vi "EMV Cold Water Check.vi"(4 "T7_DELTA_INDICATING_FLOW":dbl, 6 "Cold Water Supply Temperature":dbl, 7 "T7 Detect?":bool, 8 "error in (no error)":errorcluster, 9 "T7_DELTA_FLOW_THRESHOLD":dbl, 11 "Current T7 Temperatures":dbl[](array[numeric])) -> (0 "error out":errorcluster, 3 "T7 Detect?":bool)   [LabVIEW 2020]
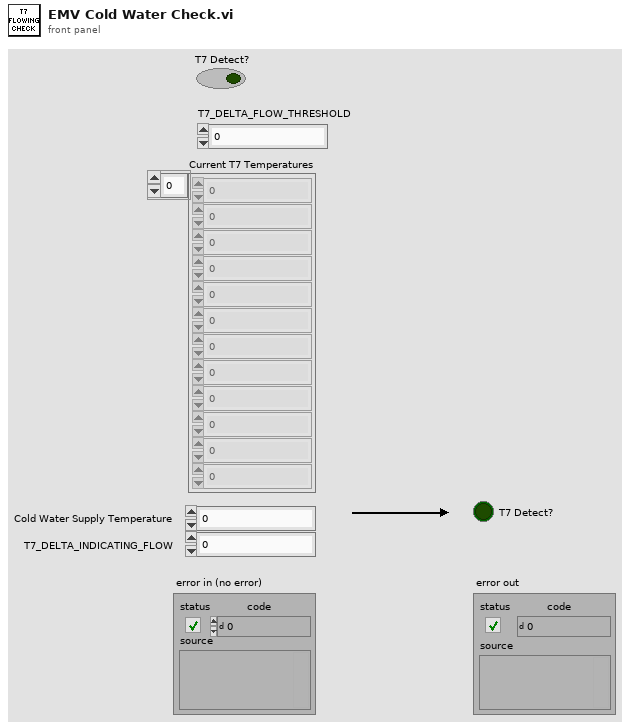
[diagram p1: front panel]
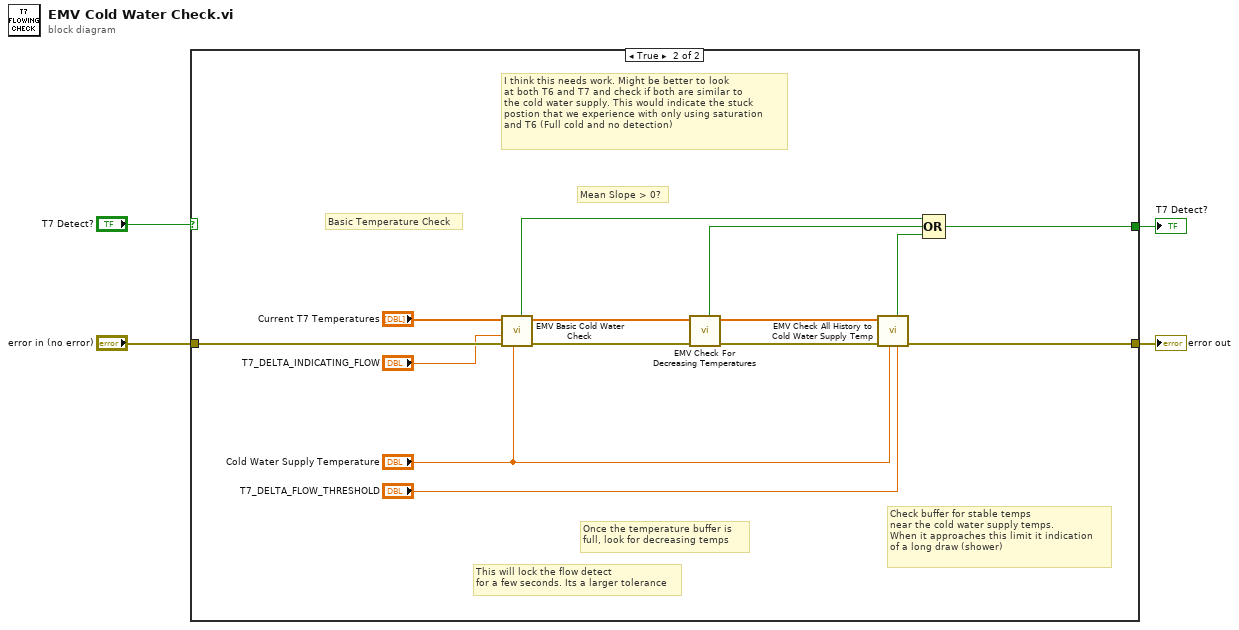
[diagram p0: block diagram]
diagram:
  n1 = case shown="True" "T7 Detect?" {
    selector: "T7 Detect?" -> [w6 _]
    tunnel: [w6 w20] -> w4
    tunnel: [w5 w19] -> w3
    tunnel: "error in (no error)" -> [w5 w18]
    frame False {
    }
    frame True {
      # "Mean Slope > 0?"
      # "Basic Temperature Check"
      # "Check buffer for stable temps \nnear the cold water supply temps.\nWhen it approaches this limit it indication\nof a long draw (shower)"
      # "Once the temperature buffer is \nfull, look for decreasing temps"
      # "This will lock the flow detect\nfor a few seconds. Its a larger tolerance"
      # "I think this needs work. Might be better to look\nat both T6 and T7 and check if both are similar to \nthe cold water supply. This would indicate the stuck\npostion that we experience with only using saturation\nand T6 (Full cold and no detection)"
      n2 = call "EMV Basic Cold Water Check.vi"("Cold Water Supply Temperature in"="Cold Water Supply Temperature", "error in (no error)"=w18, "T7_DELTA_INDICATING_FLOW"="T7_DELTA_INDICATING_FLOW", "Current T7 Temperatures in"="Current T7 Temperatures") -> ("error out"=w14:errorcluster, "Current T7 Temperatures out"=w16:dbl[], "Basic Cold Water Check"=w10:bool)  [unwired: 5 in]
      n3 = call "EMV Check For Decreasing Temperatures.vi"("error in (no error)"=w14, "Current T7 Temperatures"=w16) -> ("error out"=w13:errorcluster, "Current T7 Temperatures Output"=w11:dbl[], "Detection?"=w9:bool)  [unwired: 6 in, 1 out]
      n4 = call "EMV Check All History to Cold Water Supply Temp.vi"("T7_DELTA_FLOW_THRESHOLD"="T7_DELTA_FLOW_THRESHOLD", "Cold Water Supply Temperature"="Cold Water Supply Temperature", "error in (no error)"=w13, "Current T7 Temperatures"=w11) -> ("error out"=w19:errorcluster, "All History Is Near Supply Temp (T) = Flowing"=w8:bool)  [unwired: 6 in]
      n5 = Compound Arithmetic op=OR(w10, w9, w8) -> (w20:bool)
    }
  }
  "T7 Detect?" <- w4
  "error out" <- w3
